vi "ITask.getTaskReference.vi"(8 "error in (no error)":errorcluster, 11 "myClassIn":refnum<class "Task_BoolStopNotifier.lvclass">) -> (0 "error out":errorcluster, 2 "taskRef":refnum<vi>, 3 "myClass out":refnum<class "Task_BoolStopNotifier.lvclass">)   [LabVIEW 2023]
doc: "Returns the VI reference related to the task to handle."
uses:
  Examples/Example_Bool_Notifier_StopMech/Task_BoolStopNotifier/Task_BoolStopNotifier.lvclass
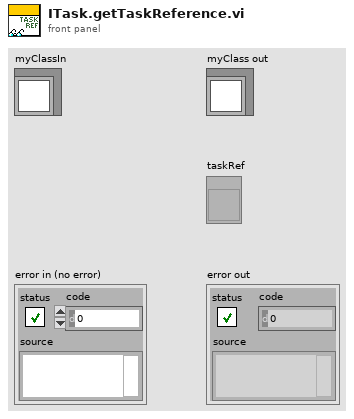
[diagram p1: front panel]
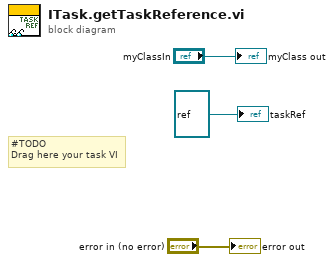
[diagram p0: block diagram]
diagram:
  # "#TODO\nDrag here your task VI"
  "error out" <- "error in (no error)"
  "myClass out" <- "myClassIn"
  "taskRef" <- refnum<vi> refnum ("taskRef")
